vi "SerialGet.vi"(8 "error in (no error)":errorcluster caption="错误输入（无错误）", 11 "serial 输入":refnum<class "serial.lvclass">) -> (0 "error out":errorcluster caption="错误输出", 2 "Serial I/O(记录)":refnum<visa-resource-name>, 3 "serial 输出":refnum<class "serial.lvclass">)   [LabVIEW 2019, in "serial.lvclass"]
uses:
  serial.lvclass
  serial.lvclass/serial.ctl
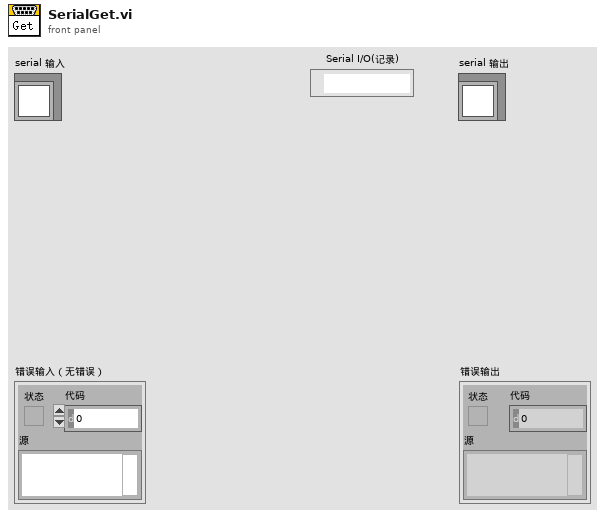
[diagram p1: front panel]
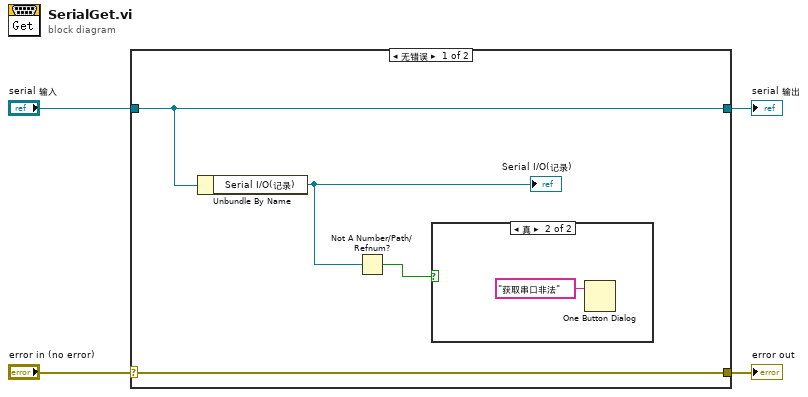
[diagram p0: block diagram]
diagram:
  n1 = case shown="无错误" "error in (no error)" {
    selector: "error in (no error)" -> [w8 w11]
    tunnel: [w8 w11] -> w3
    tunnel: [w7 w10] -> w1
    tunnel: "serial 输入" -> [w7 w10]
    frame No Error {
      n2 = Unbundle By Name(w7) -> ("Serial I/O(记录)"=w6:refnum<visa-resource-name>)
      "Serial I/O(记录)" <- w6
      n3 = Not A Number/Path/Refnum?(number/path/refnum=w6) -> (NaN/Path/Refnum?=w5:bool)
      n4 = case shown="真" w5 {
        frame False {
        }
        frame True {
          n5 = One Button Dialog(message="获取串口非法" ("消息")) -> ()  [unwired: 1 in, 1 out]
        }
      }
    }
    frame Error {
    }
  }
  "error out" <- w3
  "serial 输出" <- w1
